vi "Get Subscriptions.vi"(8 "error in (no error)":errorcluster, 11 "MQTT Server":refnum<class "Server.lvclass">) -> (0 "error out":errorcluster, 2 "Subscriptions":refnum<class "_Subscription.lvclass">[](array[class]), 3 "MQTT Server":refnum<class "Server.lvclass">)   [LabVIEW 2013, in "MQTT Server.lvlib" / "Server.lvclass"]
uses:
  Server.lvclass
  Subscription/_Subscription.lvclass
  Server.lvclass/Server.ctl
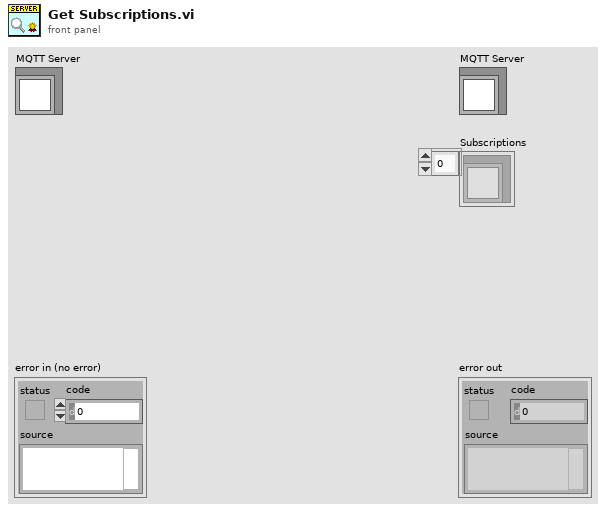
[diagram p1: front panel]
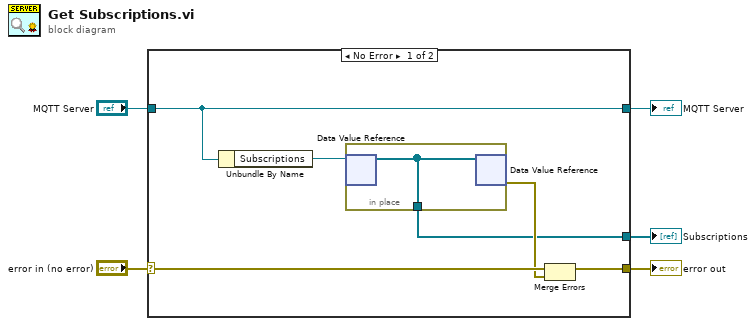
[diagram p0: block diagram]
diagram:
  n1 = case shown="No Error" "error in (no error)" {
    selector: "error in (no error)" -> [w9 w14]
    tunnel: [w7 w14] -> w4
    tunnel: [w11 w13] -> w2
    tunnel: "MQTT Server" -> [w11 w13]
    tunnel: [w6 _] -> w1
    frame No Error {
      n2 = Unbundle By Name(w11) -> ("Subscriptions"=w10:refnum<data-value>)
      n3 = in-place {
        in-place-border: [w12] -> w6
        n4 = in-place-dvr #1(w10) -> (w12:refnum<class "_Subscription.lvclass">[])  [unwired: 1 out]
        n5 = in-place-dvr #1(w12) -> (w8:errorcluster)  [unwired: 1 out]
      }
      n6 = Merge Errors(w9, w8) -> (w7:errorcluster)
    }
    frame Error {
    }
  }
  "error out" <- w4
  "MQTT Server" <- w2
  "Subscriptions" <- w1
